vi "KickOut.vi"(9 "MotorPower":dbl, 10 "Button":bool, 11 "MotorIn":dbl) -> (3 "MotorOut":dbl)   [LabVIEW 2015]
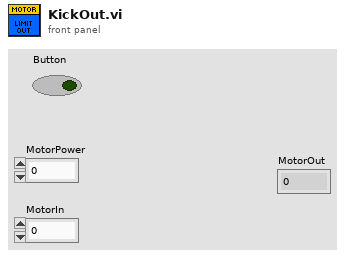
[diagram p1: front panel]
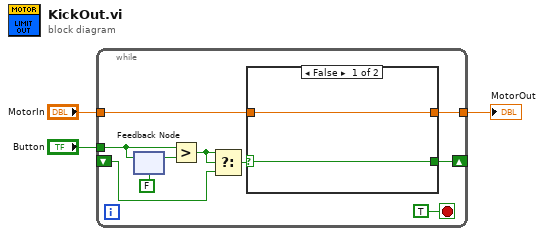
[diagram p0: block diagram]
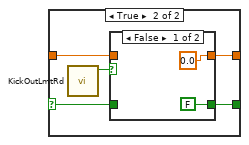
[diagram p2: hidden frame]
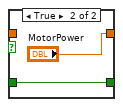
[diagram p3: hidden frame]
diagram:
  n1 = while {
    tunnel: "Button" -> [w4]
    tunnel: [w13] -> w2
    tunnel: "MotorIn" -> [w12]
    shift-right: [w6] -> _
    shift-left: _ -> [w5]
    stop <- TRUE stop-if-true
    n2 = feedback-in #1(w4) -> ()
    n3 = feedback #1(FALSE) -> (w10:bool)
    n4 = Greater?(x=w4, y=w10) -> (0:w8:bool)
    n5 = Select(t=w8, s=w8, f=w5) -> (s? t:f=w7:bool)
    n6 = case shown="False" w7 {
      selector: w7 -> [w14 w18]
      tunnel: [w15 w20] -> w13
      tunnel: w12 -> [w15 w16]
      tunnel: [w14 w17] -> w6
      frame False {
      }
      frame True {
        n7 = call "KickOutLmtRd.vi"() -> ("Pressed?"=w19:bool)  [unwired: 11 in]
        n8 = case shown="False" w19 {
          tunnel: [0.0 ("MotorIn") "MotorPower"] -> w20
          tunnel: w18 -> [_ w24]
          tunnel: [FALSE w24] -> w17
          tunnel: w16 -> [_ _]
          frame False {
          }
          frame True {
          }
        }
      }
    }
  }
  "MotorOut" <- w2
